vi "health_te.vi"(0 "teSerial":T1={"port"="COM1", "timeout"=1000, "baud"=115200, "dataBits"=8, "stopBits"=10, "flowControl"=0, "parity"=0, "termChar"=FALSE, "checkSum"=FALSE, "checkSumVal"=""} {"stopBits" items=["1.0"=10, "1.5"=15, "2.0"=20]; "parity" items=["None", "Odd", "Even", "Mark", "Space"]; "flowControl" items=["None"=0, "XON/XOFF"=1, "RTS/CTS"=2, "DTR/DSR"=4]}, 5 "Hex Address":string="00", 7 "Command":string="01", 9 "Data":string="0", 11 "Error In":errorcluster) -> (4 "Response Hex":string, 6 "Response Dec":dbl, 8 "Response":dbl, 15 "error out":errorcluster)   [LabVIEW 2018]
doc: "The Basic Serial Read and Write example performs a Serial Port Read, a Serial Port Write, or a combination of these actions. The user selects the actions (read or write) on the front panel. If both are selected, the VI will write the data first, read data, and then close the VISA session that is opened to the port. This VI will wait until the specified number of bytes is received at the port. Only the number of bytes specified will be read.\n\nINSTRUCTIONS:\n1) Select the serial resource and configuration parameters (baud rate, data bits, parity, stop bits, flow control).\n2) Select the operations to be performed. \n3) Connect the serial port to your device. If no device is available, perform a loopback test by doing one of the following. Short pins 2 and 3 on a RS-232 cable or short pin 4 to pin 8 and pin 5 to pin 9 on a RS-485/422 cable. \n4) Run the VI to see the data read. (The \"read string\" will match the \"string to write\" if a loopback test was performed.)\n\nNote: The parameters set for the serial port must match the parameters of the connected instrument or device. In this example, the bytes to read parameter specifies the number of bytes that the serial port reads. If there were more bytes at the port than the number specified in bytes to read, those bytes would not be read. Also, if you specify to read more bytes than the number of bytes actually read, you might receive a timeout error message.\n\nOn the block diagram, the Configure Serial Port VI sets the configuration parameters. The front panel displays the controls used to configure the basic parameters, such as baud rate, data bits, and parity. Constants configure the other parameters the user probably does not need set. After the VISA Configure Serial Port VI opens the VISA session and configures the port, the VI passes the VISA resource name to other VIs that perform operations on that VISA resource. The VISA Write function sends a command to the serial device and the VISA Read function returns data based on the command. The VISA Close function then closes the reference to the serial device. It is important to close the reference; otherwise communication through with that port through protocols other than VISA might not be possible."
uses:
  <vilib>/Instr/_visa.llb/VISA Configure Serial Port (Instr).vi
panel:
  out "Checksum":string
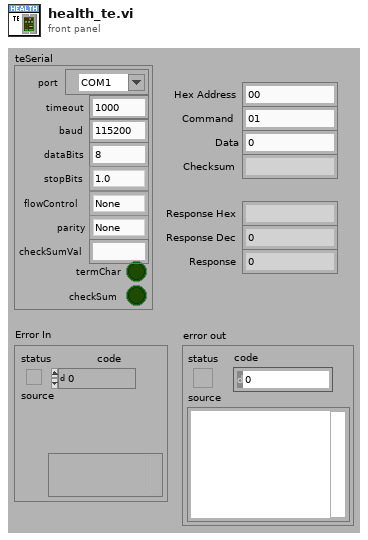
[diagram p1: front panel]
types:
  T1 = cluster{"port":refnum<visa-resource-name>, "timeout":u32, "baud":u32, "dataBits":u16, "stopBits":u16, "flowControl":u16, "parity":u16, "termChar":bool, "checkSum":bool, "checkSumVal":string}
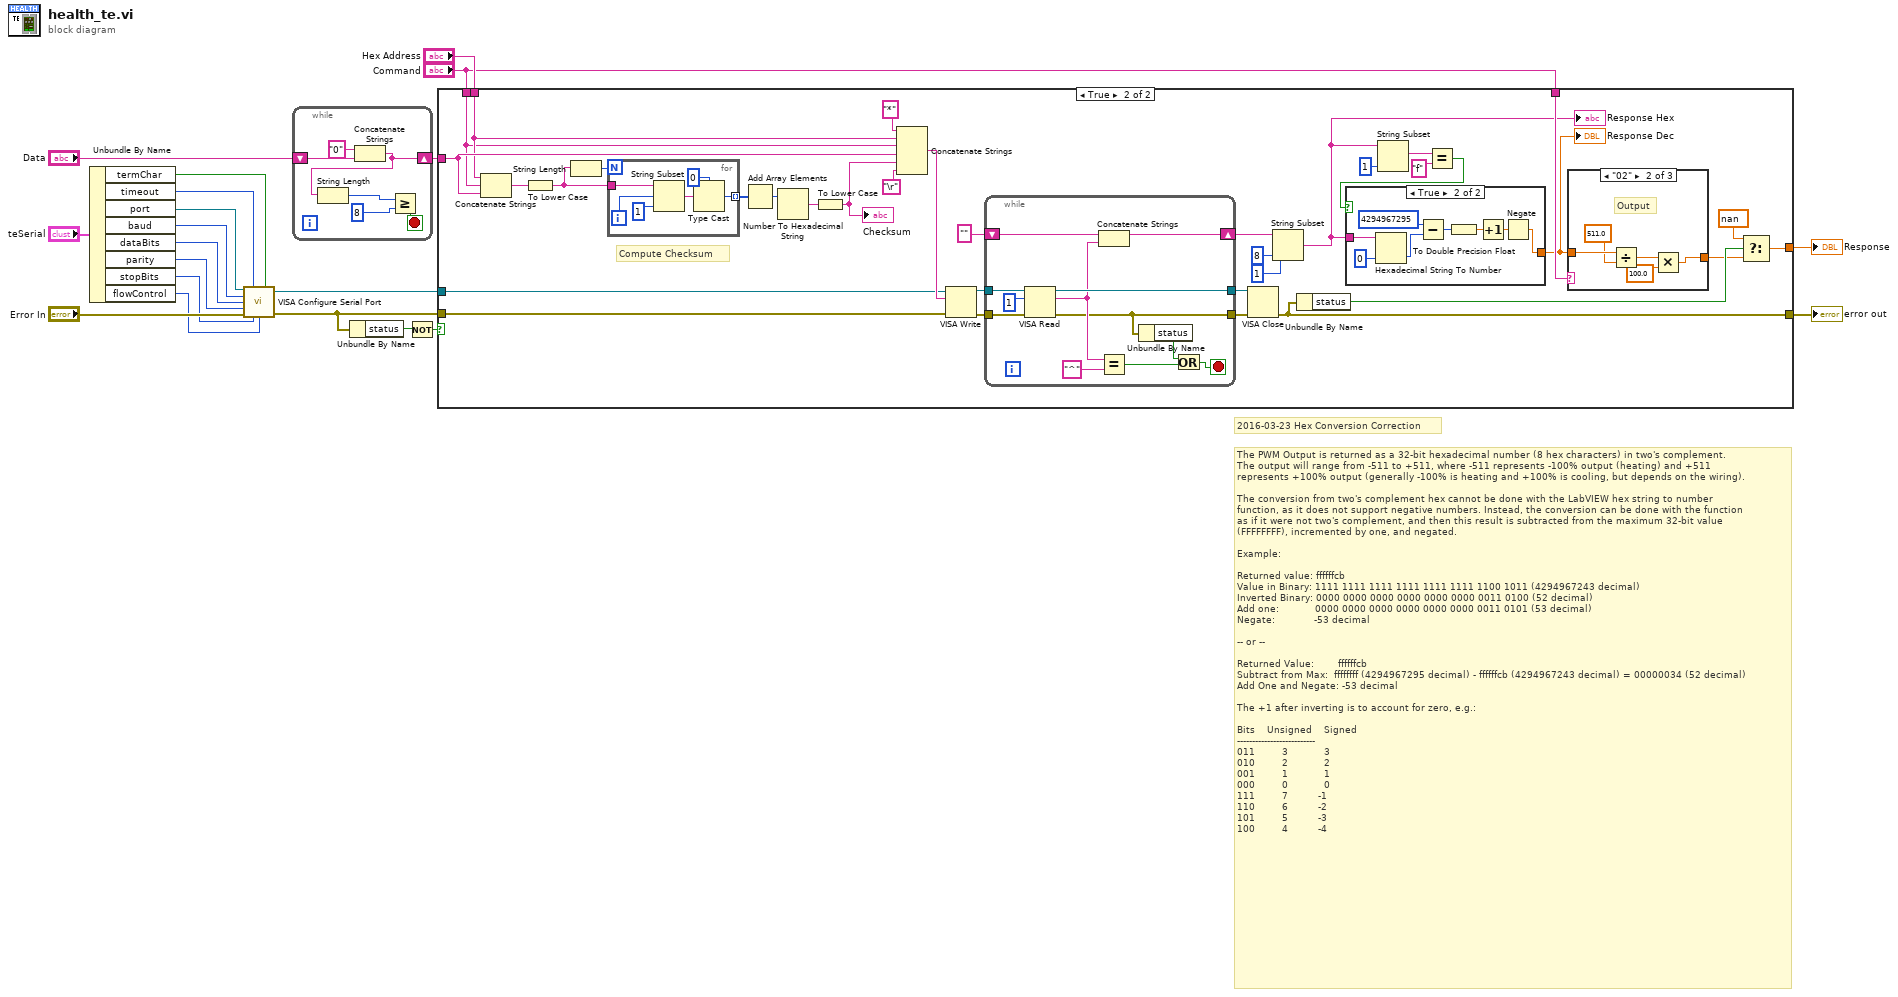
[diagram p0: block diagram]
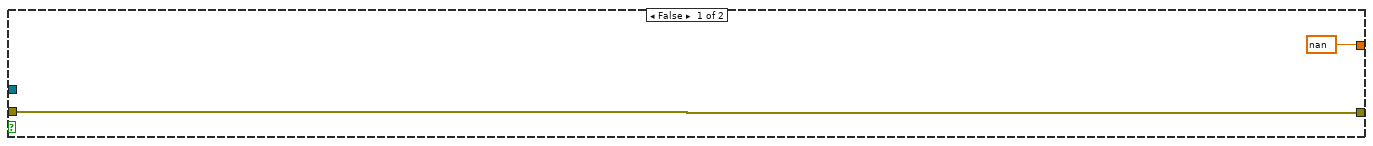
[diagram p2: hidden frame]
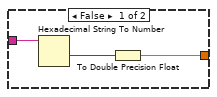
[diagram p3: hidden frame]
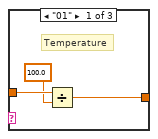
[diagram p4: hidden frame]
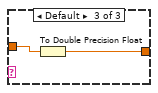
[diagram p5: hidden frame]
diagram:
  # "2016-03-23 Hex Conversion Correction"
  # "The PWM Output is returned as a 32-bit hexadecimal number (8 hex characters) in two's complement.\nThe output will range from -511 to +511, where -511 represents -100% output (heating) and +511\nrepresents +100% output (generally -100% is heating and +100% is cooling, but depends on the wiring).\n\nThe conversion from two's complement hex cannot be done with the LabVIEW hex string to number\nfunction, as it does not support negative numbers. Instead, the conversion can be done with the function\nas if it were not two's complement, and then this result is subtracted from the maximum 32-bit value\n(FFFFFFFF), incremented by one, and negated.\n\nExample:\n\nReturned value: ffffffcb\nValue in Binary: 1111 1111 1111 1111 1111 1111 1100 1011 (4294967243 decimal)\nInverted Binary: 0000 0000 0000 0000 0000 0000 0011 0100 (52 decimal)\nAdd one:            0000 0000 0000 0000 0000 0000 0011 0101 (53 decimal)\nNegate:             -53 decimal\n\n-- or --\n\nReturned Value:        ffffffcb\nSubtract from Max:  ffffffff (4294967295 decimal) - ffffffcb (4294967243 decimal) = 00000034 (52 decimal)\nAdd One and Negate: -53 decimal                \n\nThe +1 after inverting is to account for zero, e.g.:\n\nBits    Unsigned    Signed\n--------------------------\n011         3            3\n010         2            2\n001         1            1\n000         0            0\n111         7          -1\n110         6          -2\n101         5          -3\n100         4          -4"
  n1 = Unbundle By Name("teSerial") -> ("termChar"=w11:bool, "timeout"=w10:u32, "port"=w9:refnum<visa-resource-name>, "baud"=w8:u32, "dataBits"=w7:u16, "parity"=w6:u16, "stopBits"=w5:u16, "flowControl"=w4:u16)
  n2 = call-poly "VISA Configure Serial Port"("VISA resource name"=w9, "timeout (10sec)"=w10, "Enable Termination\nChar (T)"=w11, "baud rate (9600)"=w8, "data bits (8)"=w7, "parity (0:none)"=w6, "error in (no error)"="Error In", "stop bits (10: 1 bit)"=w5, "flow control (0:none)"=w4) -> ("VISA resource name out"=w19:refnum<visa-resource-name>, "error out"=w18:errorcluster)  [unwired: 5 in]
  n3 = while {
    shift-right: [w24] -> w13
    shift-left: "Data" -> [w26]
    stop <- w21 stop-if-true
    n4 = Concatenate Strings("0" ("string"), w26) -> (w24:string)
    n5 = String Length(string=w24) -> (length=w22:i32)
    n6 = Greater Or Equal?(x=w22, y=8) -> (x >= y?=w21:bool)
  }
  n7 = Unbundle By Name(w18) -> ("status"=w16:bool)
  n8 = Not(x=w16) -> (.not. x?=w17:bool)
  n9 = case shown="True" w17 {
    tunnel: w19 -> [_ w59]
    tunnel: w18 -> [w28 w58]
    tunnel: [w28 w50] -> w15
    tunnel: w13 -> [_ w40]
    tunnel: "Hex Address" -> [_ w38]
    tunnel: "Command" -> [_ w37]
    tunnel: "Command" -> [_ w36]
    tunnel: [nan ("t") w29] -> w1
    frame False {
    }
    frame True {
      # "Compute Checksum"
      n10 = Concatenate Strings(w38, w37, w40) -> (w42:string)
      n11 = To Lower Case(string=w42) -> (all lower case string=w44:string)
      n12 = String Length(string=w44) -> (length=w47:i32)
      n13 = for {
        N: w47 -> [_]
        tunnel: w44 -> [w88]
        tunnel: [w84] -> w46 mode=indexing
        i -> [w87]
        n14 = String Subset(string=w88, offset (0)=w87, length (rest)=1 ("length (rest)")) -> (substring=w85:string)
        n15 = Type Cast(type=u8 0, x=w85) -> (*(type *) &x=w84:u8)
      }
      n16 = Add Array Elements(numeric array=w46) -> (sum=w45:u8)
      n17 = Number To Hexadecimal String(2:w45) -> (0:w43:string)  [unwired: 1 in]
      n18 = To Lower Case(string=w43) -> (all lower case string=w41:string)
      "Checksum" <- w41
      n19 = Concatenate Strings("*", w38, w37, w40, w41, "\r") -> (w60:string)
      n20 = VISA Write(VISA resource name=w59, write buffer=w60, error in (no error)=w58) -> (VISA resource name out=w57:refnum<visa-resource-name>, error out=w56:errorcluster)  [unwired: 1 out]
      n21 = while {
        tunnel: [w91] -> w50
        tunnel: [w101] -> w62
        tunnel: w57 -> [w93]
        tunnel: w56 -> [w99]
        shift-right: [w97] -> w52
        shift-left: "" ("read buffer") -> [w98]
        stop <- w94 stop-if-true
        n22 = VISA Read(VISA resource name=w93, byte count=u32 1, error in (no error)=w99) -> (VISA resource name out=w101:refnum<visa-resource-name>, read buffer=w96:string, error out=w91:errorcluster)  [unwired: 1 out]
        n23 = Concatenate Strings(w98, w96) -> (w97:string)
        n24 = Equal?(x=w96, y="^") -> (x = y?=w90:bool)
        n25 = Unbundle By Name(w91) -> ("status"=w92:bool)
        n26 = Or(x=w92, y=w90) -> (x .or. y?=w94:bool)
      }
      n27 = VISA Close(VISA resource name=w62, error in (no error)=w50) -> ()  [unwired: 1 out]
      n28 = String Subset(string=w52, offset (0)=1, length (rest)=8 ("length (rest)")) -> (substring=w31:string)
      "Response Hex" <- w31
      n29 = Unbundle By Name(w50) -> ("status"=w51:bool)
      n30 = String Subset(string=w31, length (rest)=1 ("length (rest)")) -> (substring=w33:string)  [unwired: 1 in]
      n31 = Equal?(x=w33, y="f") -> (x = y?=w35:bool)
      n32 = case shown="True" w35 {
        tunnel: [w64 w68] -> w30
        tunnel: w31 -> [w65 w72]
        frame False {
          n33 = Hexadecimal String To Number(string=w65) -> (number=w63:u32)  [unwired: 2 in, 1 out]
          n34 = To Double Precision Float(number=w63) -> (double precision float=w64:dbl)
        }
        frame True {
          n35 = Hexadecimal String To Number(string=w72, default (0uL)=u32 0 ("default (0 U32)")) -> (number=w70:u32)  [unwired: 1 in, 1 out]
          n36 = Subtract(x=u32 4294967295, y=w70) -> (x-y=w69:u32)
          n37 = To Double Precision Float(number=w69) -> (double precision float=w67:dbl)
          n38 = Increment(x=w67) -> (x+1=w66:dbl)
          n39 = Negate(x=w66) -> (-x=w68:dbl)
        }
      }
      "Response Dec" <- w30
      n40 = case shown="\"02\"" w36 {
        tunnel: w30 -> [w76 w81 w82]
        tunnel: [w74 w77 w83] -> w39
        frame "01" {
          # "Temperature"
          n41 = Divide(x=w76, y=100.0) -> (x/y=w74:dbl)
        }
        frame "02" {
          # "Output"
          n42 = Divide(x=w81, y=511.0) -> (x/y=w79:dbl)
          n43 = Multiply(x=w79, y=100.0) -> (x*y=w77:dbl)
        }
        frame Default {
          n44 = To Double Precision Float(number=w82) -> (double precision float=w83:dbl)
        }
      }
      n45 = Select(t=nan, s=w51, f=w39) -> (s? t:f=w29:dbl)
    }
  }
  "error out" <- w15
  "Response" <- w1
